vi "SetHeadingLevel.vi"(8 "error in (no error)":errorcluster, 10 "HeadingLevel":T1(ring), 11 "Heading in":refnum<class "Heading.lvclass">) -> (0 "error out":errorcluster, 3 "Heading out":refnum<class "Heading.lvclass">)   [LabVIEW 2021, in "LvMarkdown.lvlib" / "Heading.lvclass"]
uses:
  Heading.lvclass
  Heading.lvclass/Heading.ctl
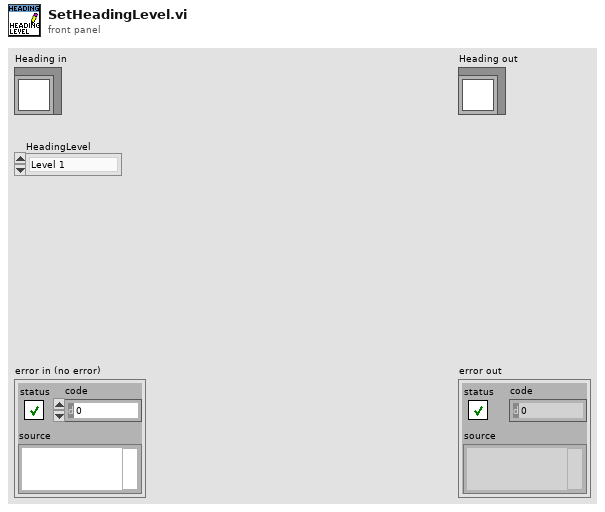
[diagram p1: front panel]
types:
  T1 = enum16{"Level 1", "Level 2", "Level 3", "Level 4", "Level 5", "Level 6"}
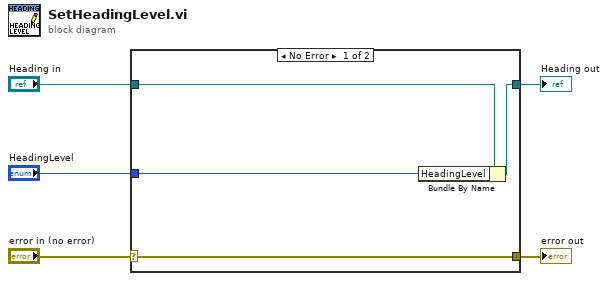
[diagram p0: block diagram]
diagram:
  n1 = case shown="No Error" "error in (no error)" {
    selector: "error in (no error)" -> [w9 w10]
    tunnel: [w9 w10] -> w4
    tunnel: [w7 w11] -> w2
    tunnel: "Heading in" -> [w8 w11]
    tunnel: "HeadingLevel" -> [w6 _]
    frame No Error {
      n2 = Bundle By Name(cluster=w8, "HeadingLevel"=w6) -> (w7:refnum<class "Heading.lvclass">)
    }
    frame Error {
    }
  }
  "error out" <- w4
  "Heading out" <- w2
